vi "testEvaluate.vi"() -> ()   [LabVIEW 2017, in "Constraint.Tests.lvlib" / "UnaryOperator.lvlib"]
uses:
  UnaryOperator.lvlib
  Constraint/Constraint/Constraint.lvclass
  Constraint/UnaryOperator/UnaryOperator.lvclass
  Assertion/Assertion.lvlib
panel:
  out "error out":errorcluster
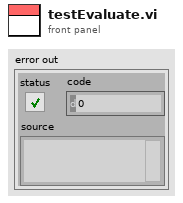
[diagram p1: front panel]
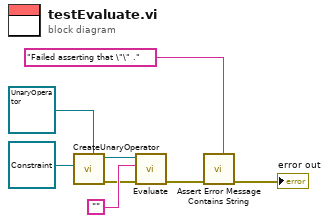
[diagram p0: block diagram]
diagram:
  n1 = call-dynamic "CreateUnaryOperator.vi"("UnaryOperator In"=refnum<class "UnaryOperator.lvclass"> refnum ("Constraint.lvlib:UnaryOperator.lvclass"), "Constraint"=refnum<class "Constraint.lvclass"> refnum ("Constraint.lvlib:Constraint.lvclass")) -> ("error out"=w3:errorcluster, "UnaryOperator"=w4:refnum<class "UnaryOperator.lvclass">)  [unwired: 8 in]
  n2 = call-dynamic "Evaluate.vi"("error in (no error)"=w3, "Actual"="", "Constraint in"=w4) -> ("error out"=w7:errorcluster)  [unwired: 7 in, 1 out]
  n3 = call "Assert Error Message Contains String.vi"("Expected"="Failed asserting that \"\" .", "error in (no error)"=w7) -> ("error out"=→"error out":errorcluster)  [unwired: 9 in]
